vi "test Float Writes to Source.vi"(8 "error in (no error)":errorcluster, 11 "TestCase in":refnum<class "Parameter Setting.lvclass">) -> (0 "error out":errorcluster, 3 "TestCase out":refnum<class "Parameter Setting.lvclass">)   [LabVIEW 2017, in "Static Errors Tests.lvlib" / "Parameter Setting.lvclass"]
uses:
  Parameter Setting.lvclass
  Parameter Setting.lvclass/Parameter Setting.ctl
  Source/VIs/Write Numeric Scalar to Source (SGL).vi
  Source/VIs/Write Numeric Scalar to Source (DBL).vi
  <vilib>/addons/_JKI Toolkits/VI Tester/TestCase.llb/TestCase.lvclass
  Source/Static Errors.lvlib
  C:/Program Files (x86)/National Instruments/LabVIEW 2017/vi.lib/addons/_JKI Toolkits/VI Tester/TestCase.llb/TestCase.lvclass
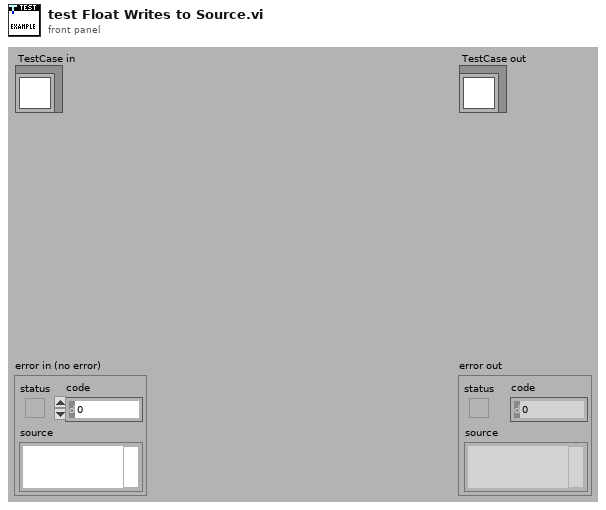
[diagram p1: front panel]
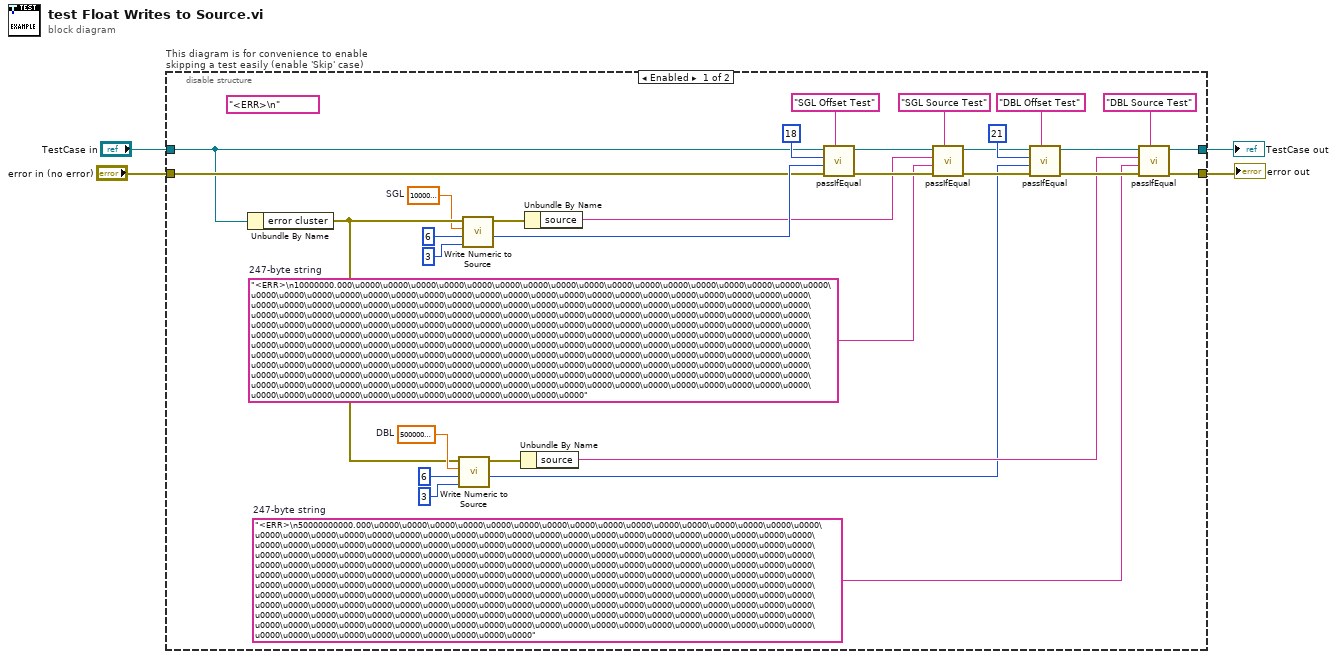
[diagram p0: block diagram]
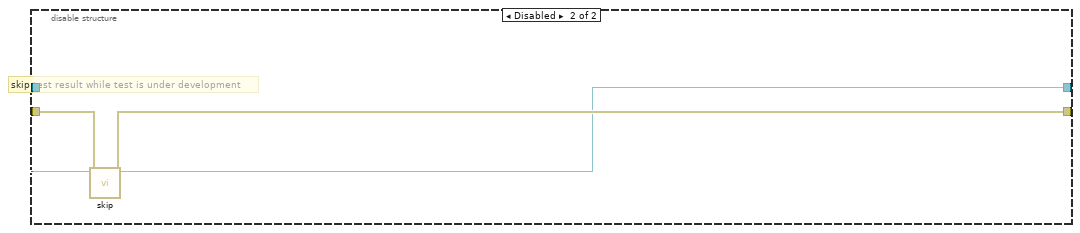
[diagram p2: hidden frame]
diagram:
  n1 = disable-structure "This diagram is for convenience to enable skipping a test easily (enable 'Skip' case)" shown="Enabled" {
    disable-tunnel: "TestCase in" -> [w10 w39]
    disable-tunnel: [w12 w37] -> w1
    disable-tunnel: [w8 w38] -> w3
    disable-tunnel: "error in (no error)" -> [w11 w36]
    frame Enabled {
      (unwired) "<ERR>\n"
      w13 = "<ERR>\n50000000000.000\u0000\u0000\u0000\u0000\u0000\u0000\u0000\u0000\u0000\u0000\u0000\u0000\u0000\u0000\u0000\u0000\u0000\u0000\u0000\u0000\u0000\u0000\u0000\u0000\u0000\u0000\u0000\u0000\u0000\u0000\u0000\u0000\u0000\u0000\u0000\u0000\u0000\u0000\u0000\u0000\u0000\u0000\u0000\u0000\u0000\u0000\u0000\u0000\u0000\u0000\u0000\u0000\u0000\u0000\u0000\u0000\u0000\u0000\u0000\u0000\u0000\u0000\u0000\u0000\u0000\u0000\u0000\u0000\u0000\u0000\u0000\u0000\u0000\u0000\u0000\u0000\u0000\u0000\u0000\u0000\u0000\u0000\u0000\u0000\u0000\u0000\u0000\u0000\u0000\u0000\u0000\u0000\u0000\u0000\u0000\u0000\u0000\u0000\u0000\u0000\u0000\u0000\u0000\u0000\u0000\u0000\u0000\u0000\u0000\u0000\u0000\u0000\u0000\u0000\u0000\u0000\u0000\u0000\u0000\u0000\u0000\u0000\u0000\u0000\u0000\u0000\u0000\u0000\u0000\u0000\u0000\u0000\u0000\u0000\u0000\u0000\u0000\u0000\u0000\u0000\u0000\u0000\u0000\u0000\u0000\u0000\u0000\u0000\u0000\u0000\u0000\u0000\u0000\u0000\u0000\u0000\u0000\u0000\u0000\u0000\u0000\u0000\u0000\u0000\u0000\u0000\u0000\u0000\u0000\u0000\u0000\u0000\u0000\u0000\u0000\u0000\u0000\u0000\u0000\u0000\u0000\u0000\u0000\u0000\u0000\u0000\u0000\u0000\u0000\u0000\u0000\u0000\u0000\u0000\u0000\u0000\u0000\u0000\u0000\u0000\u0000\u0000\u0000\u0000\u0000\u0000\u0000\u0000\u0000\u0000\u0000\u0000\u0000\u0000\u0000\u0000\u0000\u0000\u0000\u0000\u0000\u0000\u0000\u0000\u0000\u0000"  # 247-byte string
      w23 = 50000000000.0  # DBL
      w26 = "<ERR>\n10000000.000\u0000\u0000\u0000\u0000\u0000\u0000\u0000\u0000\u0000\u0000\u0000\u0000\u0000\u0000\u0000\u0000\u0000\u0000\u0000\u0000\u0000\u0000\u0000\u0000\u0000\u0000\u0000\u0000\u0000\u0000\u0000\u0000\u0000\u0000\u0000\u0000\u0000\u0000\u0000\u0000\u0000\u0000\u0000\u0000\u0000\u0000\u0000\u0000\u0000\u0000\u0000\u0000\u0000\u0000\u0000\u0000\u0000\u0000\u0000\u0000\u0000\u0000\u0000\u0000\u0000\u0000\u0000\u0000\u0000\u0000\u0000\u0000\u0000\u0000\u0000\u0000\u0000\u0000\u0000\u0000\u0000\u0000\u0000\u0000\u0000\u0000\u0000\u0000\u0000\u0000\u0000\u0000\u0000\u0000\u0000\u0000\u0000\u0000\u0000\u0000\u0000\u0000\u0000\u0000\u0000\u0000\u0000\u0000\u0000\u0000\u0000\u0000\u0000\u0000\u0000\u0000\u0000\u0000\u0000\u0000\u0000\u0000\u0000\u0000\u0000\u0000\u0000\u0000\u0000\u0000\u0000\u0000\u0000\u0000\u0000\u0000\u0000\u0000\u0000\u0000\u0000\u0000\u0000\u0000\u0000\u0000\u0000\u0000\u0000\u0000\u0000\u0000\u0000\u0000\u0000\u0000\u0000\u0000\u0000\u0000\u0000\u0000\u0000\u0000\u0000\u0000\u0000\u0000\u0000\u0000\u0000\u0000\u0000\u0000\u0000\u0000\u0000\u0000\u0000\u0000\u0000\u0000\u0000\u0000\u0000\u0000\u0000\u0000\u0000\u0000\u0000\u0000\u0000\u0000\u0000\u0000\u0000\u0000\u0000\u0000\u0000\u0000\u0000\u0000\u0000\u0000\u0000\u0000\u0000\u0000\u0000\u0000\u0000\u0000\u0000\u0000\u0000\u0000\u0000\u0000\u0000\u0000\u0000\u0000\u0000\u0000\u0000\u0000\u0000"  # 247-byte string
      w7 = sgl 10000000.0  # SGL
      n2 = Unbundle By Name(w10) -> ("error cluster"=w9:errorcluster)
      n3 = call-poly "Write Numeric to Source.vi"("precision (3)"=i16 3, "offset"=6, "value"=w23, "error in"=w9) -> ("new offset"=w14:i32, "error out"=w25:errorcluster)  [unwired: 6 in]
      n4 = call-poly "Write Numeric to Source.vi"("precision (3)"=i16 3, "offset"=6, "value"=w7, "error in"=w9) -> ("new offset"=w28:i32, "error out"=w29:errorcluster)  [unwired: 6 in]
      n5 = Unbundle By Name(w25) -> ("source"=w15:string)
      n6 = Unbundle By Name(w29) -> ("source"=w27:string)
      n7 = call-dynamic "passIfEqual.vi"("custom report message (\"\")"="SGL Offset Test" ("custom report message (\"\")"), "error in (no error)"=w11, "y"=w28, "x"=18 ("offset"), "TestCase in"=w10) -> ("error out"=w31:errorcluster, "TestCase out"=w32:refnum<class "Parameter Setting.lvclass">)  [unwired: 5 in]
      n8 = call-dynamic "passIfEqual.vi"("custom report message (\"\")"="SGL Source Test" ("custom report message (\"\")"), "error in (no error)"=w31, "y"=w26, "x"=w27, "TestCase in"=w32) -> ("error out"=w18:errorcluster, "TestCase out"=w19:refnum<class "Parameter Setting.lvclass">)  [unwired: 5 in]
      n9 = call-dynamic "passIfEqual.vi"("custom report message (\"\")"="DBL Offset Test" ("custom report message (\"\")"), "error in (no error)"=w18, "y"=w14, "x"=21 ("offset"), "TestCase in"=w19) -> ("error out"=w16:errorcluster, "TestCase out"=w22:refnum<class "Parameter Setting.lvclass">)  [unwired: 5 in]
      n10 = call-dynamic "passIfEqual.vi"("custom report message (\"\")"="DBL Source Test" ("custom report message (\"\")"), "error in (no error)"=w16, "y"=w13, "x"=w15, "TestCase in"=w22) -> ("error out"=w8:errorcluster, "TestCase out"=w12:refnum<class "Parameter Setting.lvclass">)  [unwired: 5 in]
    }
    frame Disabled {
      # "skip test result while test is under development"
      n11 = call <vilib>:"skip.vi"("error in (no error)"=w36, "TestCase in"=w39) -> ("error out"=w38:errorcluster, "TestCase out"=w37:refnum<class "Parameter Setting.lvclass">)  [unwired: 8 in]
    }
  }
  "error out" <- w3
  "TestCase out" <- w1
